vi "onAddHeader.vi"(8 "error in":errorcluster, 9 "value":string, 10 "header":string, 11 "REST Client in":refnum<class "REST Client.lvclass">) -> (0 "error out":errorcluster, 3 "REST Client out":refnum<class "REST Client.lvclass">)   [LabVIEW 2020, in "REST Client.lvlib" / "REST Client.lvclass"]
uses:
  REST Client.lvclass
  REST Client.lvclass/REST Client.ctl
  http-client-pkg/httpHeaders/httpHeaders.lvclass
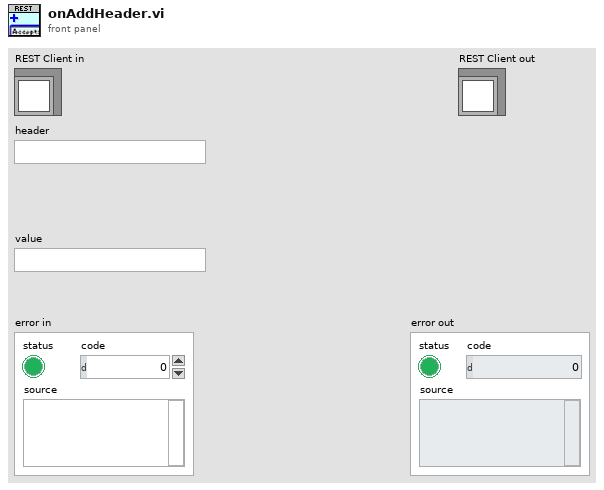
[diagram p1: front panel]
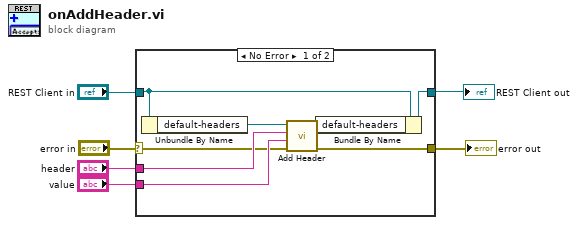
[diagram p0: block diagram]
diagram:
  n1 = case shown="No Error" "error in" {
    selector: "error in" -> [w8 w15]
    tunnel: "header" -> [w11 _]
    tunnel: "REST Client in" -> [w13 w16]
    tunnel: [w14 w16] -> w5
    tunnel: [w7 w15] -> w4
    tunnel: "value" -> [w10 _]
    frame No Error {
      n2 = Unbundle By Name(w13) -> ("default-headers"=w12:refnum<class "httpHeaders.lvclass">)
      n3 = call "Add Header.vi"("error in (no error)"=w8, "value"=w10, "header"=w11, "httpHeaders in"=w12) -> ("error out"=w7:errorcluster, "httpHeaders out"=w9:refnum<class "httpHeaders.lvclass">)  [unwired: 6 in]
      n4 = Bundle By Name(cluster=w13, "default-headers"=w9) -> (w14:refnum<class "REST Client.lvclass">)
    }
    frame Error {
    }
  }
  "error out" <- w4
  "REST Client out" <- w5
